vi "Close.vi"(8 "error in (no error)":errorcluster, 9 "Collect Timeout (-2=No collect) [-2,-1,0s,5s,10s,30s]":i32=-2, 10 "Dispose? (T)":bool=TRUE, 11 "VI Reference in":variant) -> (0 "error out":errorcluster)   [LabVIEW 2018, in "Thread.lvlib"]
uses:
  Thread.lvlib
  <vilib>/Utility/error.llb/Error Cluster From Error Code.vi
  <vilib>/ErrorRing/Error Ring.xnode
  Cache Action.ctl
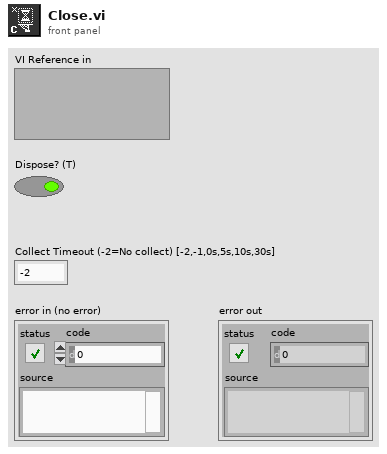
[diagram p1: front panel]
types:
  T1 = typedef "Thread.lvlib/Cache Action.ctl" = enum8{"noop", "get", "add", "remove", "remove_by_ref"}
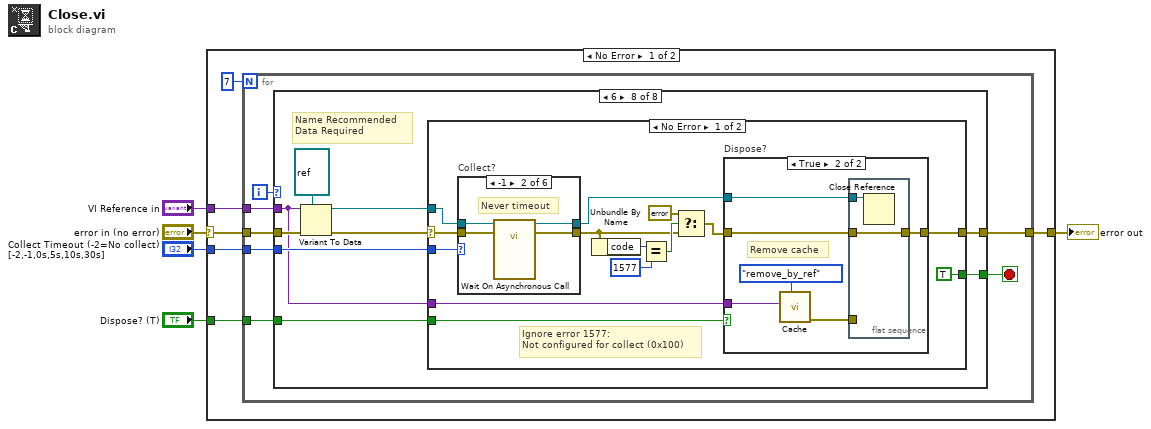
[diagram p0: block diagram]
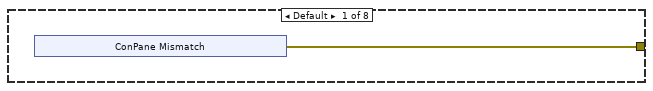
[diagram p2: hidden frame]
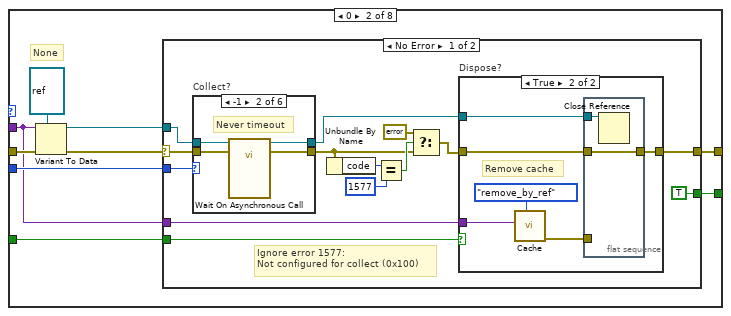
[diagram p3: hidden frame]
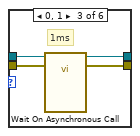
[diagram p6: hidden frame]
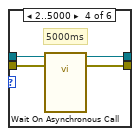
[diagram p7: hidden frame]
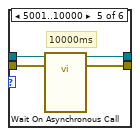
[diagram p8: hidden frame]
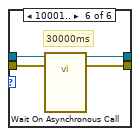
[diagram p9: hidden frame]
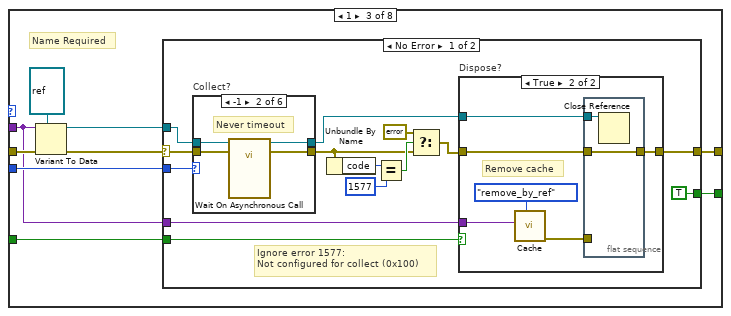
[diagram p11: hidden frame]
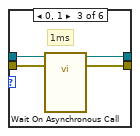
[diagram p14: hidden frame]
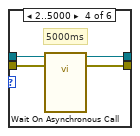
[diagram p15: hidden frame]
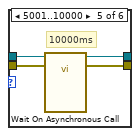
[diagram p16: hidden frame]
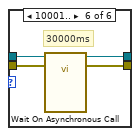
[diagram p17: hidden frame]
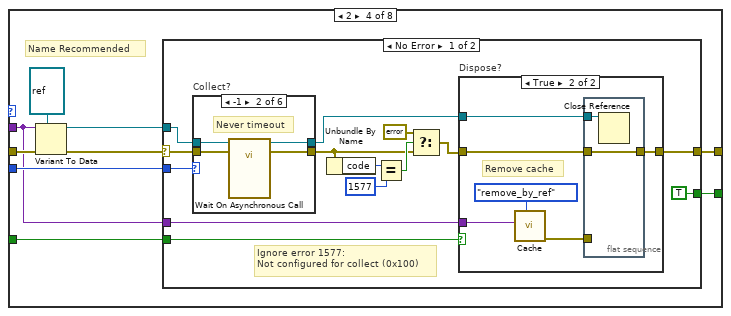
[diagram p19: hidden frame]
diagram:
  n1 = case shown="No Error" "error in (no error)" {
    selector: "error in (no error)" -> [w11 w409]
    tunnel: "VI Reference in" -> [w9 _]
    tunnel: [w6 w409] -> w4
    tunnel: "Collect Timeout (-2=No collect) [-2,-1,0s,5s,10s,30s]" -> [w8 _]
    tunnel: "Dispose? (T)" -> [w7 _]
    frame No Error {
      n2 = for {
        N: 7 -> [_]
        tunnel: w9 -> [w17]
        tunnel: w11 -> [w18]
        tunnel: [w15] -> w6
        tunnel: w8 -> [w13]
        tunnel: w7 -> [w12]
        i -> [w16]
        stop <- w14 stop-if-true
        n3 = case shown="6" w16 {
          tunnel: w18 -> [_ w32 w87 w142 w197 w252 w307 w362]
          tunnel: w17 -> [_ w24 w80 w135 w190 w245 w300 w355]
          tunnel: [w19 w29 w84 w139 w194 w249 w304 w359] -> w15
          tunnel: [_ w27 w83 w138 w193 w248 w303 w358] -> w14
          tunnel: w13 -> [_ w26 w82 w137 w192 w247 w302 w357]
          tunnel: w12 -> [_ w25 w81 w136 w191 w246 w301 w356]
          frame Default {
            n4 = xnode "ConPane Mismatch"() -> ("error out"=w19:errorcluster)
          }
          frame 0 {
            # "None"
            n5 = Variant To Data(error in=w32, type=refnum<vi> refnum ("VI Refnum"), Variant=w24) -> (data=w30:refnum<vi>, error out=w31:errorcluster)
            n6 = case shown="No Error" w31 {
              selector: w31 -> [w46 w78]
              tunnel: w30 -> [w45 _]
              tunnel: [w35 w78] -> w29
              tunnel: [TRUE _] -> w27
              tunnel: w26 -> [w43 _]
              tunnel: w25 -> [w34 _]
              tunnel: w24 -> [w33 _]
              frame No Error {
                # "Ignore error 1577:\nNot configured for collect (0x100)"
                n7 = case "Collect?" shown="-1" w43 {
                  tunnel: w46 -> [w57 w61 w65 w69 w73 w77]
                  tunnel: w45 -> [w56 w60 w64 w68 w72 w76]
                  tunnel: [w57 w59 w63 w67 w71 w75] -> w38
                  tunnel: [w56 w58 w62 w66 w70 w74] -> w42
                  frame ..-2 {
                    # "No collect"
                  }
                  frame -1 {
                    # "Never timeout"
                    n8 = call-by-ref "Wait On Asynchronous Call"(reference=w60, error in=w61) -> (reference out=w58:refnum<vi>, error out=w59:errorcluster)  [unwired: 12 in]
                  }
                  frame 0, 1 {
                    # "1ms"
                    n9 = call-by-ref "Wait On Asynchronous Call"(reference=w64, error in=w65) -> (reference out=w62:refnum<vi>, error out=w63:errorcluster)  [unwired: 12 in]
                  }
                  frame 2..5000 {
                    # "5000ms"
                    n10 = call-by-ref "Wait On Asynchronous Call"(reference=w68, error in=w69) -> (reference out=w66:refnum<vi>, error out=w67:errorcluster)  [unwired: 12 in]
                  }
                  frame 5001..10000 {
                    # "10000ms"
                    n11 = call-by-ref "Wait On Asynchronous Call"(reference=w72, error in=w73) -> (reference out=w70:refnum<vi>, error out=w71:errorcluster)  [unwired: 12 in]
                  }
                  frame 10001.. {
                    # "30000ms"
                    n12 = call-by-ref "Wait On Asynchronous Call"(reference=w76, error in=w77) -> (reference out=w74:refnum<vi>, error out=w75:errorcluster)  [unwired: 12 in]
                  }
                }
                n13 = Unbundle By Name(w38) -> ("code"=w41:i32)
                n14 = Equal?(x=w41, y=1577) -> (x = y?=w39:bool)
                n15 = Select(t=errorcluster {"status"=FALSE, "code"=0, "source"=""}, s=w39, f=w38) -> (s? t:f=w36:errorcluster)
                n16 = case "Dispose?" shown="True" w34 {
                  tunnel: w42 -> [_ w52]
                  tunnel: w36 -> [w47 w49]
                  tunnel: [w47 w48] -> w35
                  tunnel: w33 -> [_ w53]
                  frame False {
                  }
                  frame True {
                    # "Remove cache"
                    n17 = call "Cache.vi"("Action"=Cache_Action."remove_by_ref", "VI in"=w53) -> ("error out"=w50:errorcluster)  [unwired: 5 in, 4 out]
                    n18 = flat-sequence {
                      tunnel: w52 -> [w55]
                      tunnel: w50 -> [_]
                      tunnel: w49 -> [w54]
                      tunnel: [w54] -> w48
                      frame #0 {
                        n19 = Close Reference(reference=w55) -> ()  [unwired: 1 in, 1 out]
                      }
                    }
                  }
                }
              }
              frame Error {
              }
            }
          }
          frame 1 {
            # "Name Required"
            n20 = Variant To Data(error in=w87, type=refnum<vi> refnum ("VI Refnum"), Variant=w80) -> (data=w85:refnum<vi>, error out=w86:errorcluster)
            n21 = case shown="No Error" w86 {
              selector: w86 -> [w101 w133]
              tunnel: w85 -> [w100 _]
              tunnel: [w90 w133] -> w84
              tunnel: [TRUE _] -> w83
              tunnel: w82 -> [w98 _]
              tunnel: w81 -> [w89 _]
              tunnel: w80 -> [w88 _]
              frame No Error {
                # "Ignore error 1577:\nNot configured for collect (0x100)"
                n22 = case "Collect?" shown="-1" w98 {
                  tunnel: w101 -> [w112 w116 w120 w124 w128 w132]
                  tunnel: w100 -> [w111 w115 w119 w123 w127 w131]
                  tunnel: [w112 w114 w118 w122 w126 w130] -> w93
                  tunnel: [w111 w113 w117 w121 w125 w129] -> w97
                  frame ..-2 {
                    # "No collect"
                  }
                  frame -1 {
                    # "Never timeout"
                    n23 = call-by-ref "Wait On Asynchronous Call"(reference=w115, error in=w116) -> (reference out=w113:refnum<vi>, error out=w114:errorcluster)  [unwired: 12 in]
                  }
                  frame 0, 1 {
                    # "1ms"
                    n24 = call-by-ref "Wait On Asynchronous Call"(reference=w119, error in=w120) -> (reference out=w117:refnum<vi>, error out=w118:errorcluster)  [unwired: 12 in]
                  }
                  frame 2..5000 {
                    # "5000ms"
                    n25 = call-by-ref "Wait On Asynchronous Call"(reference=w123, error in=w124) -> (reference out=w121:refnum<vi>, error out=w122:errorcluster)  [unwired: 12 in]
                  }
                  frame 5001..10000 {
                    # "10000ms"
                    n26 = call-by-ref "Wait On Asynchronous Call"(reference=w127, error in=w128) -> (reference out=w125:refnum<vi>, error out=w126:errorcluster)  [unwired: 12 in]
                  }
                  frame 10001.. {
                    # "30000ms"
                    n27 = call-by-ref "Wait On Asynchronous Call"(reference=w131, error in=w132) -> (reference out=w129:refnum<vi>, error out=w130:errorcluster)  [unwired: 12 in]
                  }
                }
                n28 = Unbundle By Name(w93) -> ("code"=w96:i32)
                n29 = Equal?(x=w96, y=1577) -> (x = y?=w94:bool)
                n30 = Select(t=errorcluster {"status"=FALSE, "code"=0, "source"=""}, s=w94, f=w93) -> (s? t:f=w91:errorcluster)
                n31 = case "Dispose?" shown="True" w89 {
                  tunnel: w97 -> [_ w107]
                  tunnel: w91 -> [w102 w104]
                  tunnel: [w102 w103] -> w90
                  tunnel: w88 -> [_ w108]
                  frame False {
                  }
                  frame True {
                    # "Remove cache"
                    n32 = call "Cache.vi"("Action"=Cache_Action."remove_by_ref", "VI in"=w108) -> ("error out"=w105:errorcluster)  [unwired: 5 in, 4 out]
                    n33 = flat-sequence {
                      tunnel: w107 -> [w110]
                      tunnel: w105 -> [_]
                      tunnel: w104 -> [w109]
                      tunnel: [w109] -> w103
                      frame #0 {
                        n34 = Close Reference(reference=w110) -> ()  [unwired: 1 in, 1 out]
                      }
                    }
                  }
                }
              }
              frame Error {
              }
            }
          }
          frame 2 {
            # "Name Recommended"
            n35 = Variant To Data(error in=w142, type=refnum<vi> refnum ("VI Refnum"), Variant=w135) -> (data=w140:refnum<vi>, error out=w141:errorcluster)
            n36 = case shown="No Error" w141 {
              selector: w141 -> [w156 w188]
              tunnel: w140 -> [w155 _]
              tunnel: [w145 w188] -> w139
              tunnel: [TRUE _] -> w138
              tunnel: w137 -> [w153 _]
              tunnel: w136 -> [w144 _]
              tunnel: w135 -> [w143 _]
              frame No Error {
                # "Ignore error 1577:\nNot configured for collect (0x100)"
                n37 = case "Collect?" shown="-1" w153 {
                  tunnel: w156 -> [w167 w171 w175 w179 w183 w187]
                  tunnel: w155 -> [w166 w170 w174 w178 w182 w186]
                  tunnel: [w167 w169 w173 w177 w181 w185] -> w148
                  tunnel: [w166 w168 w172 w176 w180 w184] -> w152
                  frame ..-2 {
                    # "No collect"
                  }
                  frame -1 {
                    # "Never timeout"
                    n38 = call-by-ref "Wait On Asynchronous Call"(reference=w170, error in=w171) -> (reference out=w168:refnum<vi>, error out=w169:errorcluster)  [unwired: 12 in]
                  }
                  frame 0, 1 {
                    # "1ms"
                    n39 = call-by-ref "Wait On Asynchronous Call"(reference=w174, error in=w175) -> (reference out=w172:refnum<vi>, error out=w173:errorcluster)  [unwired: 12 in]
                  }
                  frame 2..5000 {
                    # "5000ms"
                    n40 = call-by-ref "Wait On Asynchronous Call"(reference=w178, error in=w179) -> (reference out=w176:refnum<vi>, error out=w177:errorcluster)  [unwired: 12 in]
                  }
                  frame 5001..10000 {
                    # "10000ms"
                    n41 = call-by-ref "Wait On Asynchronous Call"(reference=w182, error in=w183) -> (reference out=w180:refnum<vi>, error out=w181:errorcluster)  [unwired: 12 in]
                  }
                  frame 10001.. {
                    # "30000ms"
                    n42 = call-by-ref "Wait On Asynchronous Call"(reference=w186, error in=w187) -> (reference out=w184:refnum<vi>, error out=w185:errorcluster)  [unwired: 12 in]
                  }
                }
                n43 = Unbundle By Name(w148) -> ("code"=w151:i32)
                n44 = Equal?(x=w151, y=1577) -> (x = y?=w149:bool)
                n45 = Select(t=errorcluster {"status"=FALSE, "code"=0, "source"=""}, s=w149, f=w148) -> (s? t:f=w146:errorcluster)
                n46 = case "Dispose?" shown="True" w144 {
                  tunnel: w152 -> [_ w162]
                  tunnel: w146 -> [w157 w159]
                  tunnel: [w157 w158] -> w145
                  tunnel: w143 -> [_ w163]
                  frame False {
                  }
                  frame True {
                    # "Remove cache"
                    n47 = call "Cache.vi"("Action"=Cache_Action."remove_by_ref", "VI in"=w163) -> ("error out"=w160:errorcluster)  [unwired: 5 in, 4 out]
                    n48 = flat-sequence {
                      tunnel: w162 -> [w165]
                      tunnel: w160 -> [_]
                      tunnel: w159 -> [w164]
                      tunnel: [w164] -> w158
                      frame #0 {
                        n49 = Close Reference(reference=w165) -> ()  [unwired: 1 in, 1 out]
                      }
                    }
                  }
                }
              }
              frame Error {
              }
            }
          }
          frame 3 {
            # "Name Required\nData Required"
            n50 = Variant To Data(error in=w197, type=refnum<vi> refnum ("VI Refnum"), Variant=w190) -> (data=w195:refnum<vi>, error out=w196:errorcluster)
            n51 = case shown="No Error" w196 {
              selector: w196 -> [w211 w243]
              tunnel: w195 -> [w210 _]
              tunnel: [w200 w243] -> w194
              tunnel: [TRUE _] -> w193
              tunnel: w192 -> [w208 _]
              tunnel: w191 -> [w199 _]
              tunnel: w190 -> [w198 _]
              frame No Error {
                # "Ignore error 1577:\nNot configured for collect (0x100)"
                n52 = case "Collect?" shown="-1" w208 {
                  tunnel: w211 -> [w222 w226 w230 w234 w238 w242]
                  tunnel: w210 -> [w221 w225 w229 w233 w237 w241]
                  tunnel: [w222 w224 w228 w232 w236 w240] -> w203
                  tunnel: [w221 w223 w227 w231 w235 w239] -> w207
                  frame ..-2 {
                    # "No collect"
                  }
                  frame -1 {
                    # "Never timeout"
                    n53 = call-by-ref "Wait On Asynchronous Call"(reference=w225, error in=w226) -> (reference out=w223:refnum<vi>, error out=w224:errorcluster)  [unwired: 12 in]
                  }
                  frame 0, 1 {
                    # "1ms"
                    n54 = call-by-ref "Wait On Asynchronous Call"(reference=w229, error in=w230) -> (reference out=w227:refnum<vi>, error out=w228:errorcluster)  [unwired: 12 in]
                  }
                  frame 2..5000 {
                    # "5000ms"
                    n55 = call-by-ref "Wait On Asynchronous Call"(reference=w233, error in=w234) -> (reference out=w231:refnum<vi>, error out=w232:errorcluster)  [unwired: 12 in]
                  }
                  frame 5001..10000 {
                    # "10000ms"
                    n56 = call-by-ref "Wait On Asynchronous Call"(reference=w237, error in=w238) -> (reference out=w235:refnum<vi>, error out=w236:errorcluster)  [unwired: 12 in]
                  }
                  frame 10001.. {
                    # "30000ms"
                    n57 = call-by-ref "Wait On Asynchronous Call"(reference=w241, error in=w242) -> (reference out=w239:refnum<vi>, error out=w240:errorcluster)  [unwired: 12 in]
                  }
                }
                n58 = Unbundle By Name(w203) -> ("code"=w206:i32)
                n59 = Equal?(x=w206, y=1577) -> (x = y?=w204:bool)
                n60 = Select(t=errorcluster {"status"=FALSE, "code"=0, "source"=""}, s=w204, f=w203) -> (s? t:f=w201:errorcluster)
                n61 = case "Dispose?" shown="True" w199 {
                  tunnel: w207 -> [_ w217]
                  tunnel: w201 -> [w212 w214]
                  tunnel: [w212 w213] -> w200
                  tunnel: w198 -> [_ w218]
                  frame False {
                  }
                  frame True {
                    # "Remove cache"
                    n62 = call "Cache.vi"("Action"=Cache_Action."remove_by_ref", "VI in"=w218) -> ("error out"=w215:errorcluster)  [unwired: 5 in, 4 out]
                    n63 = flat-sequence {
                      tunnel: w217 -> [w220]
                      tunnel: w215 -> [_]
                      tunnel: w214 -> [w219]
                      tunnel: [w219] -> w213
                      frame #0 {
                        n64 = Close Reference(reference=w220) -> ()  [unwired: 1 in, 1 out]
                      }
                    }
                  }
                }
              }
              frame Error {
              }
            }
          }
          frame 4 {
            # "Name Recommended\nData Recommended"
            n65 = Variant To Data(error in=w252, type=refnum<vi> refnum ("VI Refnum"), Variant=w245) -> (data=w250:refnum<vi>, error out=w251:errorcluster)
            n66 = case shown="No Error" w251 {
              selector: w251 -> [w266 w298]
              tunnel: w250 -> [w265 _]
              tunnel: [w255 w298] -> w249
              tunnel: [TRUE _] -> w248
              tunnel: w247 -> [w263 _]
              tunnel: w246 -> [w254 _]
              tunnel: w245 -> [w253 _]
              frame No Error {
                # "Ignore error 1577:\nNot configured for collect (0x100)"
                n67 = case "Collect?" shown="-1" w263 {
                  tunnel: w266 -> [w277 w281 w285 w289 w293 w297]
                  tunnel: w265 -> [w276 w280 w284 w288 w292 w296]
                  tunnel: [w277 w279 w283 w287 w291 w295] -> w258
                  tunnel: [w276 w278 w282 w286 w290 w294] -> w262
                  frame ..-2 {
                    # "No collect"
                  }
                  frame -1 {
                    # "Never timeout"
                    n68 = call-by-ref "Wait On Asynchronous Call"(reference=w280, error in=w281) -> (reference out=w278:refnum<vi>, error out=w279:errorcluster)  [unwired: 12 in]
                  }
                  frame 0, 1 {
                    # "1ms"
                    n69 = call-by-ref "Wait On Asynchronous Call"(reference=w284, error in=w285) -> (reference out=w282:refnum<vi>, error out=w283:errorcluster)  [unwired: 12 in]
                  }
                  frame 2..5000 {
                    # "5000ms"
                    n70 = call-by-ref "Wait On Asynchronous Call"(reference=w288, error in=w289) -> (reference out=w286:refnum<vi>, error out=w287:errorcluster)  [unwired: 12 in]
                  }
                  frame 5001..10000 {
                    # "10000ms"
                    n71 = call-by-ref "Wait On Asynchronous Call"(reference=w292, error in=w293) -> (reference out=w290:refnum<vi>, error out=w291:errorcluster)  [unwired: 12 in]
                  }
                  frame 10001.. {
                    # "30000ms"
                    n72 = call-by-ref "Wait On Asynchronous Call"(reference=w296, error in=w297) -> (reference out=w294:refnum<vi>, error out=w295:errorcluster)  [unwired: 12 in]
                  }
                }
                n73 = Unbundle By Name(w258) -> ("code"=w261:i32)
                n74 = Equal?(x=w261, y=1577) -> (x = y?=w259:bool)
                n75 = Select(t=errorcluster {"status"=FALSE, "code"=0, "source"=""}, s=w259, f=w258) -> (s? t:f=w256:errorcluster)
                n76 = case "Dispose?" shown="True" w254 {
                  tunnel: w262 -> [_ w272]
                  tunnel: w256 -> [w267 w269]
                  tunnel: [w267 w268] -> w255
                  tunnel: w253 -> [_ w273]
                  frame False {
                  }
                  frame True {
                    # "Remove cache"
                    n77 = call "Cache.vi"("Action"=Cache_Action."remove_by_ref", "VI in"=w273) -> ("error out"=w270:errorcluster)  [unwired: 5 in, 4 out]
                    n78 = flat-sequence {
                      tunnel: w272 -> [w275]
                      tunnel: w270 -> [_]
                      tunnel: w269 -> [w274]
                      tunnel: [w274] -> w268
                      frame #0 {
                        n79 = Close Reference(reference=w275) -> ()  [unwired: 1 in, 1 out]
                      }
                    }
                  }
                }
              }
              frame Error {
              }
            }
          }
          frame 5 {
            # "Name Required\nData Recommended"
            n80 = Variant To Data(error in=w307, type=refnum<vi> refnum ("VI Refnum"), Variant=w300) -> (data=w305:refnum<vi>, error out=w306:errorcluster)
            n81 = case shown="No Error" w306 {
              selector: w306 -> [w321 w353]
              tunnel: w305 -> [w320 _]
              tunnel: [w310 w353] -> w304
              tunnel: [TRUE _] -> w303
              tunnel: w302 -> [w318 _]
              tunnel: w301 -> [w309 _]
              tunnel: w300 -> [w308 _]
              frame No Error {
                # "Ignore error 1577:\nNot configured for collect (0x100)"
                n82 = case "Collect?" shown="-1" w318 {
                  tunnel: w321 -> [w332 w336 w340 w344 w348 w352]
                  tunnel: w320 -> [w331 w335 w339 w343 w347 w351]
                  tunnel: [w332 w334 w338 w342 w346 w350] -> w313
                  tunnel: [w331 w333 w337 w341 w345 w349] -> w317
                  frame ..-2 {
                    # "No collect"
                  }
                  frame -1 {
                    # "Never timeout"
                    n83 = call-by-ref "Wait On Asynchronous Call"(reference=w335, error in=w336) -> (reference out=w333:refnum<vi>, error out=w334:errorcluster)  [unwired: 12 in]
                  }
                  frame 0, 1 {
                    # "1ms"
                    n84 = call-by-ref "Wait On Asynchronous Call"(reference=w339, error in=w340) -> (reference out=w337:refnum<vi>, error out=w338:errorcluster)  [unwired: 12 in]
                  }
                  frame 2..5000 {
                    # "5000ms"
                    n85 = call-by-ref "Wait On Asynchronous Call"(reference=w343, error in=w344) -> (reference out=w341:refnum<vi>, error out=w342:errorcluster)  [unwired: 12 in]
                  }
                  frame 5001..10000 {
                    # "10000ms"
                    n86 = call-by-ref "Wait On Asynchronous Call"(reference=w347, error in=w348) -> (reference out=w345:refnum<vi>, error out=w346:errorcluster)  [unwired: 12 in]
                  }
                  frame 10001.. {
                    # "30000ms"
                    n87 = call-by-ref "Wait On Asynchronous Call"(reference=w351, error in=w352) -> (reference out=w349:refnum<vi>, error out=w350:errorcluster)  [unwired: 12 in]
                  }
                }
                n88 = Unbundle By Name(w313) -> ("code"=w316:i32)
                n89 = Equal?(x=w316, y=1577) -> (x = y?=w314:bool)
                n90 = Select(t=errorcluster {"status"=FALSE, "code"=0, "source"=""}, s=w314, f=w313) -> (s? t:f=w311:errorcluster)
                n91 = case "Dispose?" shown="True" w309 {
                  tunnel: w317 -> [_ w327]
                  tunnel: w311 -> [w322 w324]
                  tunnel: [w322 w323] -> w310
                  tunnel: w308 -> [_ w328]
                  frame False {
                  }
                  frame True {
                    # "Remove cache"
                    n92 = call "Cache.vi"("Action"=Cache_Action."remove_by_ref", "VI in"=w328) -> ("error out"=w325:errorcluster)  [unwired: 5 in, 4 out]
                    n93 = flat-sequence {
                      tunnel: w327 -> [w330]
                      tunnel: w325 -> [_]
                      tunnel: w324 -> [w329]
                      tunnel: [w329] -> w323
                      frame #0 {
                        n94 = Close Reference(reference=w330) -> ()  [unwired: 1 in, 1 out]
                      }
                    }
                  }
                }
              }
              frame Error {
              }
            }
          }
          frame 6 {
            # "Name Recommended\nData Required"
            n95 = Variant To Data(error in=w362, type=refnum<vi> refnum ("VI Refnum"), Variant=w355) -> (data=w360:refnum<vi>, error out=w361:errorcluster)
            n96 = case shown="No Error" w361 {
              selector: w361 -> [w376 w408]
              tunnel: w360 -> [w375 _]
              tunnel: [w365 w408] -> w359
              tunnel: [TRUE _] -> w358
              tunnel: w357 -> [w373 _]
              tunnel: w356 -> [w364 _]
              tunnel: w355 -> [w363 _]
              frame No Error {
                # "Ignore error 1577:\nNot configured for collect (0x100)"
                n97 = case "Collect?" shown="-1" w373 {
                  tunnel: w376 -> [w387 w391 w395 w399 w403 w407]
                  tunnel: w375 -> [w386 w390 w394 w398 w402 w406]
                  tunnel: [w387 w389 w393 w397 w401 w405] -> w368
                  tunnel: [w386 w388 w392 w396 w400 w404] -> w372
                  frame ..-2 {
                    # "No collect"
                  }
                  frame -1 {
                    # "Never timeout"
                    n98 = call-by-ref "Wait On Asynchronous Call"(reference=w390, error in=w391) -> (reference out=w388:refnum<vi>, error out=w389:errorcluster)  [unwired: 12 in]
                  }
                  frame 0, 1 {
                    # "1ms"
                    n99 = call-by-ref "Wait On Asynchronous Call"(reference=w394, error in=w395) -> (reference out=w392:refnum<vi>, error out=w393:errorcluster)  [unwired: 12 in]
                  }
                  frame 2..5000 {
                    # "5000ms"
                    n100 = call-by-ref "Wait On Asynchronous Call"(reference=w398, error in=w399) -> (reference out=w396:refnum<vi>, error out=w397:errorcluster)  [unwired: 12 in]
                  }
                  frame 5001..10000 {
                    # "10000ms"
                    n101 = call-by-ref "Wait On Asynchronous Call"(reference=w402, error in=w403) -> (reference out=w400:refnum<vi>, error out=w401:errorcluster)  [unwired: 12 in]
                  }
                  frame 10001.. {
                    # "30000ms"
                    n102 = call-by-ref "Wait On Asynchronous Call"(reference=w406, error in=w407) -> (reference out=w404:refnum<vi>, error out=w405:errorcluster)  [unwired: 12 in]
                  }
                }
                n103 = Unbundle By Name(w368) -> ("code"=w371:i32)
                n104 = Equal?(x=w371, y=1577) -> (x = y?=w369:bool)
                n105 = Select(t=errorcluster {"status"=FALSE, "code"=0, "source"=""}, s=w369, f=w368) -> (s? t:f=w366:errorcluster)
                n106 = case "Dispose?" shown="True" w364 {
                  tunnel: w372 -> [_ w382]
                  tunnel: w366 -> [w377 w379]
                  tunnel: [w377 w378] -> w365
                  tunnel: w363 -> [_ w383]
                  frame False {
                  }
                  frame True {
                    # "Remove cache"
                    n107 = call "Cache.vi"("Action"=Cache_Action."remove_by_ref", "VI in"=w383) -> ("error out"=w380:errorcluster)  [unwired: 5 in, 4 out]
                    n108 = flat-sequence {
                      tunnel: w382 -> [w385]
                      tunnel: w380 -> [_]
                      tunnel: w379 -> [w384]
                      tunnel: [w384] -> w378
                      frame #0 {
                        n109 = Close Reference(reference=w385) -> ()  [unwired: 1 in, 1 out]
                      }
                    }
                  }
                }
              }
              frame Error {
              }
            }
          }
        }
      }
    }
    frame Error {
    }
  }
  "error out" <- w4
